vi "Convert AIM Time Stamp to NI Time Stamp.vi"(11 "IRIG Time Stamp":T1={"Days of year"=1, "Hours"=0, "Minutes"=0, "Seconds"=0, "Milliseconds"=0}) -> (3 "Time Stamp":timestamp format="%<%.6X\n%x>T")   [LabVIEW 2020]
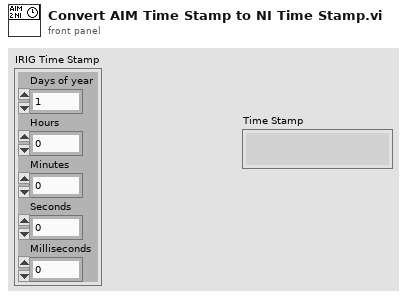
[diagram p1: front panel]
types:
  T1 = cluster{"Days of year":u32, "Hours":u32, "Minutes":u32, "Seconds":u32, "Milliseconds":u32}
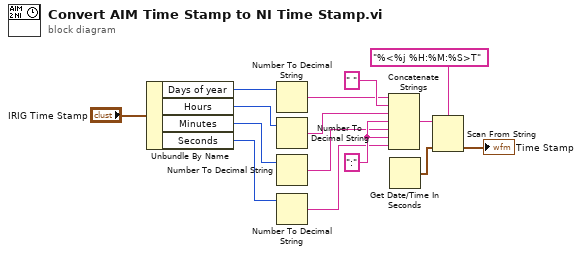
[diagram p0: block diagram]
diagram:
  w13 = ":"
  n1 = Unbundle By Name("IRIG Time Stamp") -> ("Days of year"=w5:u32, "Hours"=w6:u32, "Minutes"=w7:u32, "Seconds"=w8:u32)
  n2 = Number To Decimal String(number=w5) -> (decimal integer string=w9:string)  [unwired: 1 in]
  n3 = Number To Decimal String(number=w6) -> (decimal integer string=w10:string)  [unwired: 1 in]
  n4 = Number To Decimal String(number=w7) -> (decimal integer string=w11:string)  [unwired: 1 in]
  n5 = Number To Decimal String(number=w8) -> (decimal integer string=w12:string)  [unwired: 1 in]
  n6 = Concatenate Strings(w9, " " ("string"), w10, w13, w11, w13, w12) -> (w15:string)
  n7 = Get Date/Time In Seconds() -> (seconds since 1Jan1904=w1:timestamp)
  n8 = Scan From String(format string="%<%j %H:%M:%S>T", input string=w15, default 1=w1) -> (output 1=→"Time Stamp":timestamp)  [unwired: 2 in, 3 out]
